vi "Calculate Derivative.vi"(9 "Chart":refnum<vi>, 11 "Viscosity":dbl) -> (3 "Cluster":cluster{"dx/dt":dbl, "dx/dt":dbl})   [LabVIEW 2019, in "SME_Data_Acquisition.lvlib"]
uses:
  SME_Data_Acquisition.lvlib
  <vilib>/ptbypt/NI_PtbyPt.lvlib
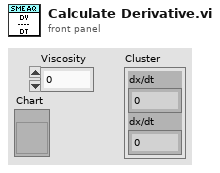
[diagram p1: front panel]
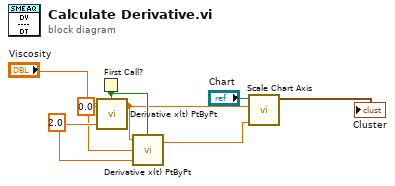
[diagram p0: block diagram]
diagram:
  w7 = 0.0 ("initial condition")
  w8 = 2.0 ("dt")
  n1 = First Call?() -> (First Call?: T/F=w6:bool)
  n2 = call <vilib>:"Derivative x(t) PtByPt.vi"("initialize"=w6, "dt"=w8, "initial condition"=w7, "x"="Viscosity") -> ("dx/dt"=w4:dbl)  [unwired: 1 out]
  n3 = call <vilib>:"Derivative x(t) PtByPt.vi"("initialize"=w6, "dt"=w8, "initial condition"=w7, "x"=w4) -> ("dx/dt"=w3:dbl)  [unwired: 1 out]
  n4 = call "Scale Chart Axis.vi"("V2"=w3, "V1"=w4, "Chart"="Chart") -> ("Chart"=→"Cluster":cluster{"Viscosity":dbl, "Temperature":dbl})  [unwired: 8 in]
